vi "BuildMenu5.vi"(0 "XRef":T15, 1 "MenuRef":T14, 2 "Point":T12, 3 "Menu Type":T11, 4 "State In":T2) -> (14 "Fatal Error Out":T1)   [LabVIEW 2020, in "FlexBlock.xnode"]
uses:
  FlexBlock.xnode
  <vilib>/XNodeSupport/XNodeXNodeRef.ctl
  <vilib>/XNodeSupport/XNodeMenuRef.ctl
  <vilib>/XNodeSupport/XNodePoint.ctl
  <vilib>/XNodeSupport/XNodeInt.ctl
  <vilib>/XNodeSupport/XNodeMenuType.ctl
  State.ctl
  FlexBlocks/Type Descriptor.ctl
  FlexBlocks/Terminal Direction.ctl
  FlexBlocks/Value Mode.ctl
  FlexBlocks/Terminal State.ctl
  FlexBlocks/Special Terminal.ctl
  FlexBlocks/Errors.ctl
  <vilib>/picture/picture.llb/imagedata.ctl
  FlexBlocks/Calculated Sizes.ctl
  <vilib>/XNodeSupport/XNodeErrorCluster.ctl
  <vilib>/XNodeSupport/NI_XNodeSupport.lvlib
  FlexBlocks/FlexBlocks.lvlib
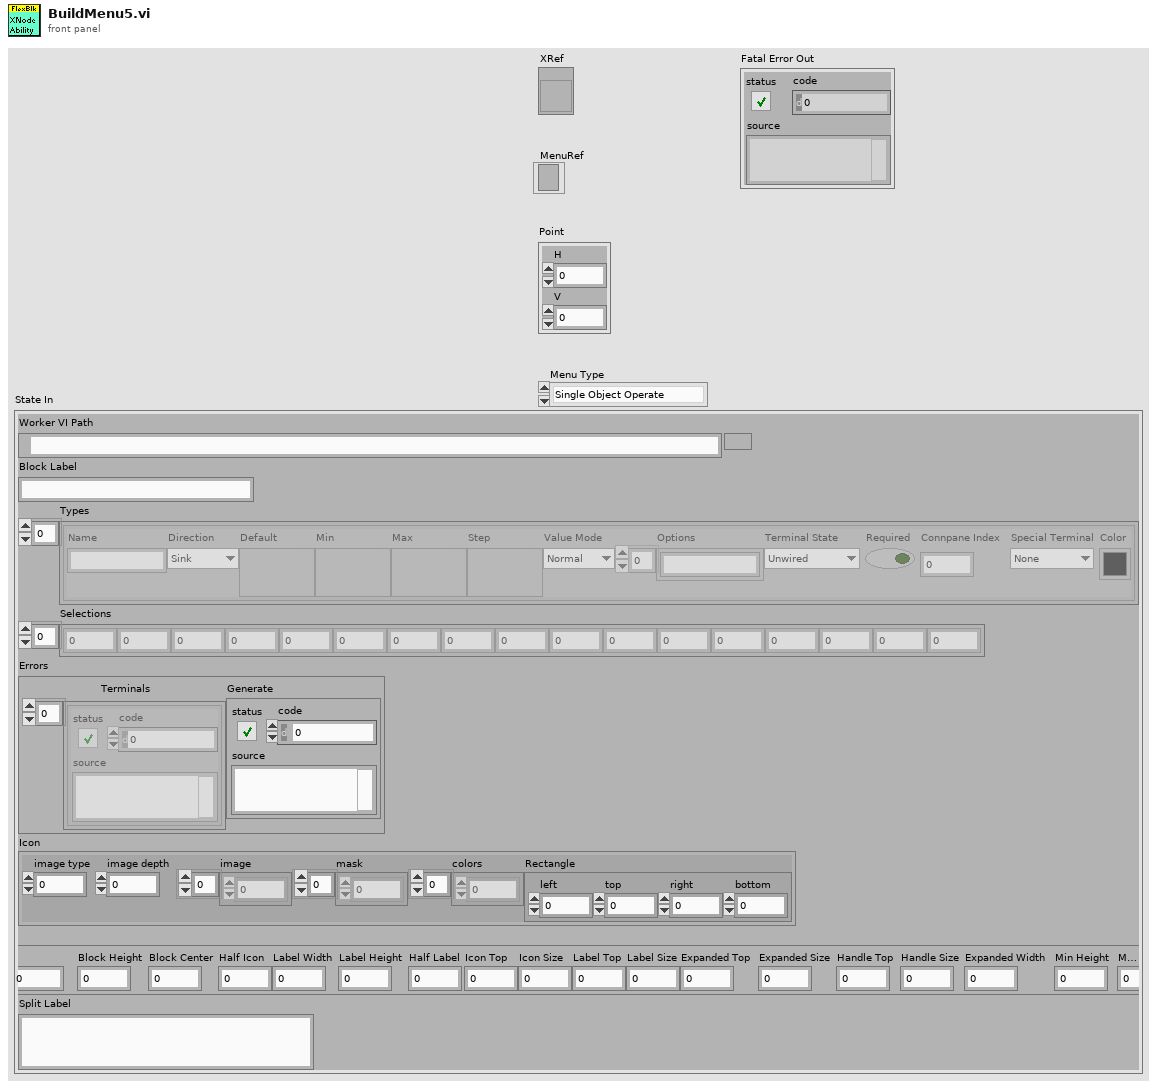
[diagram p1: front panel]
types:
  T1 = typedef "NI_XNodeSupport.lvlib/XNodeErrorCluster.ctl" = errorcluster
  T2 = typedef "FlexBlock.xnode/State.ctl" = cluster{"Worker VI Path":path, "Block Label":string, "Types":T3[], "Selections":i32[], "Errors":T8, "Icon":T9, "Calcd Sizes":T10, "Split Label":string}
  T3 = typedef "FlexBlocks.lvlib/Type Descriptor.ctl" = cluster{"Name":string, "Direction":T4, "Default":variant, "Min":variant, "Max":variant, "Step":variant, "Value Mode":T5, "Options":string[], "Terminal State":T6, "Required":bool, "Connpane Index":i32, "Special Terminal":T7, "Color":u32}
  T4 = typedef "FlexBlocks.lvlib/Terminal Direction.ctl" = enum16{"Sink", "Source"}
  T5 = typedef "FlexBlocks.lvlib/Value Mode.ctl" = enum16{"Normal", "Range", "Select"}
  T6 = typedef "FlexBlocks.lvlib/Terminal State.ctl" = enum16{"Unwired", "BadType", "BadRef", "Channel", "Value", "Control Ref"}
  T7 = typedef "FlexBlocks.lvlib/Special Terminal.ctl" = enum16{"None", "Action", "Init", "Tag", "State in", "State out", "Error"}
  T8 = typedef "FlexBlocks.lvlib/Errors.ctl" = cluster{"Terminals":errorcluster[], "Generate":errorcluster}
  T9 = typedef "imagedata.ctl" = cluster{"image type":i32, "image depth":i32, "image":u8[], "mask":u8[], "colors":u32[], "Rectangle":cluster{"left":i16, "top":i16, "right":i16, "bottom":i16}}
  T10 = typedef "FlexBlocks.lvlib/Calculated Sizes.ctl" = cluster{"Text Width":i32, "Text Height":i32, "Half Text":i32, "Block Width":i32, "Block Height":i32, "Block Center":i32, "Half Icon":i32, "Label Width":i32, "Label Height":i32, "Half Label":i32, "Icon Top":i32, "Icon Size":i32, "Label Top":i32, "Label Size":i32, "Expanded Top":i32, "Expanded Size":i32, "Handle Top":i32, "Handle Size":i32, "Expanded Width":i32, "Min Height":i32, "Max Height":i32}
  T11 = typedef "NI_XNodeSupport.lvlib/XNodeMenuType.ctl" = enum32{"Single Object Operate", "Single Object Popup", "Multi Object Popup Master", "Multi Object Popup Other"}
  T12 = typedef "NI_XNodeSupport.lvlib/XNodePoint.ctl" = cluster{"H":T13, "V":T13}
  T13 = typedef "NI_XNodeSupport.lvlib/XNodeInt.ctl" = i32
  T14 = typedef "NI_XNodeSupport.lvlib/XNodeMenuRef.ctl" = refnum<k9>
  T15 = typedef "NI_XNodeSupport.lvlib/XNodeXNodeRef.ctl" = refnum<vi>
  T16 = typedef "FlexBlocks.lvlib/Size Constants.ctl" = cluster{"Icon":i32, "Value Width":i32, "BG Rounding":i32, "Term Width":i32, "Term Height":i32, "Text Offset":i32, "Value Padding":i32, "Select Padding":i32, "Min Block Width":i32, "Vertical Margin":i32, "Size Handle Height":i32, "Name Padding":i32, "Collapsed Spacing":i32}
  T17 = cluster{"left":i16, "top":i16, "right":i16, "bottom":i16}
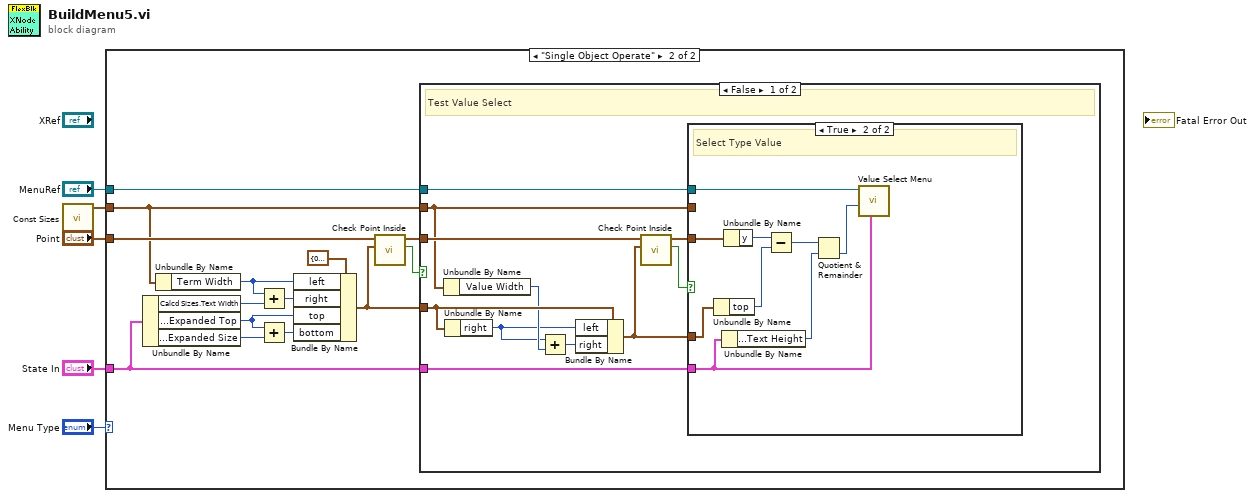
[diagram p0: block diagram]
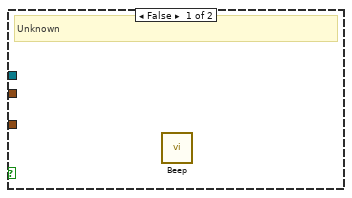
[diagram p3: hidden frame]
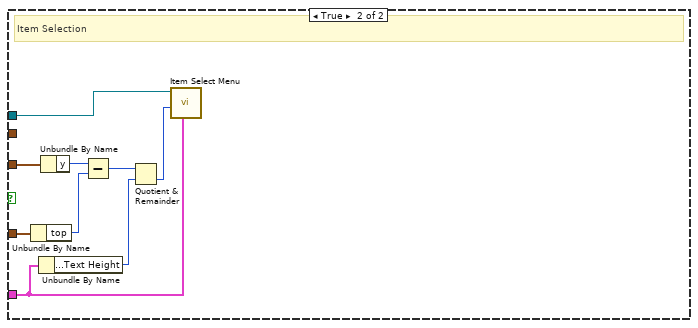
[diagram p4: hidden frame]
diagram:
  n1 = call "Const Sizes.vi"() -> ("Sizes"=w1:T16)  [unwired: 11 in]
  n2 = case shown="\"Single Object Operate\"" "Menu Type" {
    tunnel: "Point" -> [_ w12]
    tunnel: "State In" -> [_ w8]
    tunnel: "MenuRef" -> [_ w6]
    tunnel: w1 -> [_ w7]
    frame Default {
    }
    frame "Single Object Operate" {
      n3 = Unbundle By Name(w8) -> ("Calcd Sizes.Text Width"=w17:i32, "Calcd Sizes.Expanded Top"=w14:i32, "Calcd Sizes.Expanded Size"=w15:i32)
      n4 = Unbundle By Name(w7) -> ("Term Width"=w16:i32)
      n5 = Add(x=w16, y=w17) -> (x+y=w18:i32)
      n6 = Add(x=w14, y=w15) -> (x+y=w13:i32)
      n7 = Bundle By Name(cluster=T17 {"left"=0, "top"=0, "right"=0, "bottom"=0} ("rect"), "left"=w16, "right"=w18, "top"=w14, "bottom"=w13) -> (w9:T17)
      n8 = call "Check Point Inside.vi"("rect"=w9, "Point In"=w12) -> ("Inside"=w11:bool, "Point"=w10:cluster{"x":T13, "y":T13})  [unwired: 8 in]
      n9 = case shown="False" w11 {
        tunnel: w10 -> [w26 w46]
        tunnel: w9 -> [w30 w47]
        tunnel: w8 -> [w21 w42]
        tunnel: w7 -> [w25 _]
        tunnel: w6 -> [w20 w48]
        frame False {
          # "Test Value Select"
          n10 = Unbundle By Name(w25) -> ("Value Width"=w29:i32)
          n11 = Unbundle By Name(w30) -> ("right"=w27:i16)
          n12 = Add(x=w27, y=w29) -> (x+y=w28:i32)
          n13 = Bundle By Name(cluster=w30, "left"=w27, "right"=w28) -> (w22:T17)
          n14 = call "Check Point Inside.vi"("rect"=w22, "Point In"=w26) -> ("Inside"=w23:bool, "Point"=w24:cluster{"x":T13, "y":T13})  [unwired: 8 in]
          n15 = case shown="True" w23 {
            tunnel: w25 -> [_ _]
            tunnel: w24 -> [_ w34]
            tunnel: w22 -> [_ w35]
            tunnel: w21 -> [_ w31]
            tunnel: w20 -> [_ w33]
            frame False {
              # "Unknown"
              n16 = call <vilib>:"Beep.vi"() -> ()  [unwired: 12 in]
            }
            frame True {
              # "Select Type Value"
              n17 = Unbundle By Name(w35) -> ("top"=w38:i16)
              n18 = Unbundle By Name(w31) -> ("Calcd Sizes.Text Height"=w36:i32)
              n19 = Unbundle By Name(w34) -> ("y"=w39:T13)
              n20 = Subtract(x=w39, y=w38) -> (x-y=w37:T13)
              n21 = Quotient & Remainder(x=w37, y=w36) -> (floor(x/y)=w32:T13)  [unwired: 1 out]
              n22 = call "Value Select Menu.vi"("State"=w31, "Index"=w32, "MenuRef"=w33) -> ()  [unwired: 9 in]
            }
          }
        }
        frame True {
          # "Item Selection"
          n23 = Unbundle By Name(w47) -> ("top"=w44:i16)
          n24 = Unbundle By Name(w42) -> ("Calcd Sizes.Text Height"=w41:i32)
          n25 = Unbundle By Name(w46) -> ("y"=w45:T13)
          n26 = Subtract(x=w45, y=w44) -> (x-y=w43:T13)
          n27 = Quotient & Remainder(x=w43, y=w41) -> (floor(x/y)=w40:T13)  [unwired: 1 out]
          n28 = call "Item Select Menu.vi"("State"=w42, "Index"=w40, "MenuRef"=w48) -> ()  [unwired: 9 in]
        }
      }
    }
  }
